vi "ElectrodesLabelsToPickeringChannels.vi"(8 "error in (no error)":errorcluster, 9 "Labels":u16[](array[ring]) items=["", "I+", "I-", "V1", "V2", "V3", "Vsg"], 10 "Electrodes":T1(array[ring]), 11 "Control Experiment in":refnum<class "Control Experiment.lvclass">) -> (0 "error out":errorcluster, 1 "Y Channel Array":string[][](array[string]), 2 "X Channel Array":string[](array[string]), 3 "Control Experiment out":refnum<class "Control Experiment.lvclass">)   [LabVIEW 2019, in "Control Experiment.lvclass"]
uses:
  Control Experiment.lvclass
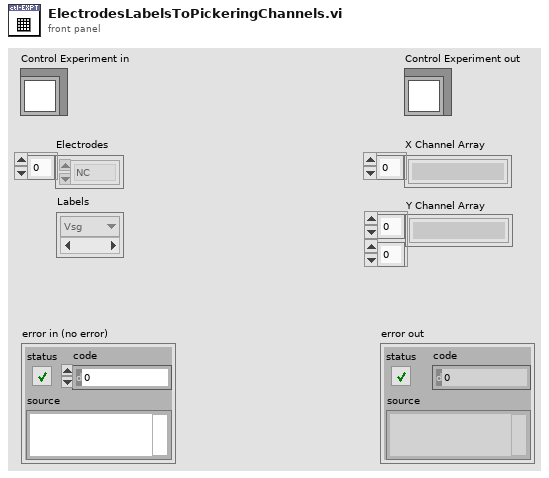
[diagram p1: front panel]
types:
  T1 = enum16{"NC", "26", "27", "28", "1", "2", "3", "4", "5", "6", "7", "8", "9", "10", "11", "12", "13", "14", "15", "16", "17", "18", "19", "20", "21", "22", "23", "24", "25"}[]
  T2 = cluster{"x config":cluster{"Electrode":enum16{"NC", "26", "27", "28", "1", "2", "3", "4", "5", "6", "7", "8", "9", "10", "11", "12", "13", "14", "15", "16", "17", "18", "19", "20", "21", "22", "23", "24", "25"}[], "X Channels":string[]}, "y config":cluster{"Label":u16[], "Y Channels":string[][]}}
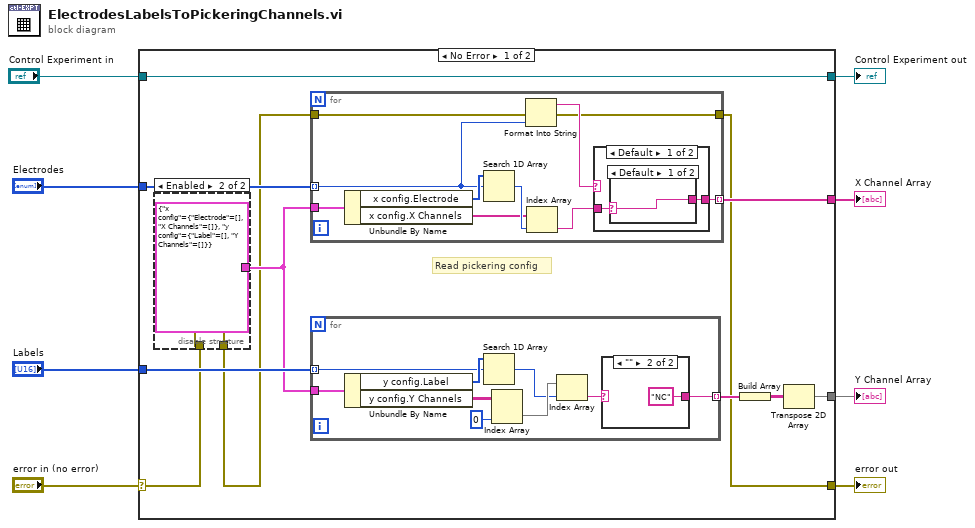
[diagram p0: block diagram]
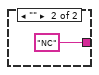
[diagram p4: hidden frame]
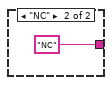
[diagram p5: hidden frame]
diagram:
  n1 = case shown="No Error" "error in (no error)" {
    selector: "error in (no error)" -> [w10 w51]
    tunnel: "Electrodes" -> [w19 _]
    tunnel: [w18 _] -> w7
    tunnel: "Labels" -> [w17 _]
    tunnel: [w12 w51] -> w5
    tunnel: [w11 _] -> w4
    tunnel: [w9 w50] -> w2
    tunnel: "Control Experiment in" -> [w9 w50]
    frame No Error {
      # "Read pickering config"
      n2 = disable-structure shown="Enabled" {
        disable-tunnel: [_ T2 {"x config"={"Electrode"=[], "X Channels"=[]}, "y config"={"Label"=[], "Y Channels"=[]}} ("Pickering Config")] -> w14
        disable-tunnel: [w21 w23] -> w13
        disable-tunnel: w10 -> [w20 w23]
        frame Disabled {
        }
        frame Enabled {
        }
      }
      n3 = for {
        tunnel: [w40] -> w18 mode=indexing
        tunnel: w14 -> [w43]
        tunnel: w19 -> [w39] mode=indexing
        tunnel: w13 -> [w36]
        tunnel: [w35] -> w12
        n4 = Unbundle By Name(w43) -> ("x config.Electrode"=w42:T1, "x config.X Channels"=w41:string[])
        n5 = Search 1D Array(1D array=w42, element=w39) -> (index of element=w44:i32)  [unwired: 1 in]
        n6 = Format Into String(error in=w36, w39) -> (resulting string=w37:string, error out=w35:errorcluster)  [unwired: 2 in]
        n7 = Index Array(array=w41, index=w44) -> (element=w38:string)
        n8 = case shown="Default" w37 {
          tunnel: [w45 "NC"] -> w40
          tunnel: w38 -> [w46 _]
          frame Default {
            n9 = case shown="Default" w46 {
              selector: w46 -> [w47 _]
              tunnel: [w47 "NC"] -> w45
              frame Default {
              }
              frame "" {
              }
            }
          }
          frame "NC" {
          }
        }
      }
      n10 = for {
        tunnel: w14 -> [w32]
        tunnel: w17 -> [w30] mode=indexing
        tunnel: [w24] -> w16 mode=indexing
        n11 = Unbundle By Name(w32) -> ("y config.Label"=w31:u16[], "y config.Y Channels"=w28:string[][])
        n12 = Search 1D Array(1D array=w31, element=w30) -> (index of element=w25:i32)  [unwired: 1 in]
        n13 = Index Array(array=w28, index (col)=0 ("disabled index (col)")) -> (element=w26:string[])  [unwired: 1 in]
        n14 = Index Array(array=w26, index=w25) -> (element=w27:string)
        n15 = case shown="\"\"" w27 {
          selector: w27 -> [w33 _]
          tunnel: [w33 "NC"] -> w24
          frame Default {
          }
          frame "" {
          }
        }
      }
      n16 = Build Array(w16) -> (w15:string[][])
      n17 = Transpose 2D Array(2D array=w15) -> (transposed array=w11:string[][])
    }
    frame Error {
    }
  }
  "error out" <- w5
  "X Channel Array" <- w7
  "Y Channel Array" <- w4
  "Control Experiment out" <- w2
